vi "CG test stand DAQ main V2.vi"() -> ()   [LabVIEW 2020]
doc: "This example demonstrates how to read N channels of analog input from a LINX device."
uses:
  <vilib>/MakerHub/LINX/LMH-LINX.lvlib
  <vilib>/MakerHub/LINX/Public/Peripherals/Analog/Analog Read N Chans.vi
  <vilib>/MakerHub/LINX/Public/Utilities/Open Serial.vi
  <vilib>/Analysis/Matrix/NI_Matrix.lvlib
  <vilib>/Utility/file.llb/Write Delimited Spreadsheet (DBL).vi
  <vilib>/Analysis/Matrix/Numeric/Conversions/Array To Matrix - RA.vi
panel:
  in  "?":T1(tab)
  out "?":string
  out "?":string
  out "?":string
  out "?":string
  out "?":string
  out "?":string
  out "?":string
  out "?":dbl
  out "?":dbl
  out "?":dbl
  out "?":dbl
  out "?":dbl
  out "?":dbl
  out "?":dbl
  in  "Serial Port":refnum<visa-resource-name>
  in  "Filename":string
  in  "File extension":string
  in  "Path":path
  out "Full filepath":string
  out "error out":errorcluster
  out "?":dbl
  out "?":dbl
  out "?":dbl
  out "?":dbl
  out "?":dbl
  out "?":dbl
  out "?":dbl
  out "?":dbl
  out "?":dbl
  out "?":dbl
  out "?":dbl
  out "?":dbl
  out "?":dbl
  out "?":dbl
  out "?":dbl
  out "?":dbl
  out "?":dbl
  out "?":dbl
  out "?":dbl
  out "?":dbl
  out "?":dbl
  out "?":dbl
  out "?":dbl
  out "?":dbl
  out "?":dbl
  out "?":dbl
  out "?":dbl
  out "?":dbl
  out "?":dbl
  out "?":dbl
  out "?":dbl
  out "?":dbl
  out "?":dbl
  out "?":dbl
  out "?":dbl
  out "?":dbl
  out "?":dbl
  out "?":dbl
  out "?":dbl
  out "?":dbl
  out "?":dbl
  out "?":dbl
  out "?":dbl
  out "?":dbl
  out "?":dbl
  out "?":dbl
  out "?":dbl
  out "?":dbl
  out "?":dbl
  out "?":string
  out "?":dbl
  out "?":dbl
  out "?":dbl
  out "?":dbl
  out "?":dbl
  out "?":dbl
  out "?":dbl
  out "?":dbl
  out "?":dbl
  out "?":dbl
  out "?":dbl
  out "?":dbl
  out "?":dbl
  out "?":dbl
  out "?":string
  out "?":string
  out "?":dbl
  out "?":dbl
  out "?":dbl
  out "?":dbl
  out "?":dbl
  out "?":dbl
  out "?":dbl
  out "?":string
  out "?":dbl
  out "?":dbl
  out "?":dbl
  out "?":dbl
  out "?":dbl
  out "?":dbl
  out "?":dbl
  out "?":string
  in  "+      B":dbl
  in  "AX":dbl
  in  "Analog Port":dbl
  out "Time Stamp":timestamp
  out "Voltage":dbl
  out "Voltage":dbl(graph)
  out "Filtered Voltage":dbl(graph)
  out "Unfiltered Voltage":dbl
  out "Filtered Voltage":dbl
  out "Loop Rate (Hz)":u32
  in  "Stop Button":bool
  out "Pressure":dbl(graph)
  out "Pressure (PSI)":dbl
  out "WRITING TO FILE":bool
  in  "?":bool
  # "File Writing"
  # "Analog Inputs"
  # "Analog Port"
  # "Voltage In"
  # "X3"
  # "X2"
  # "X1"
  # "B"
  # "Instrument name"
  # "Scaled Value"
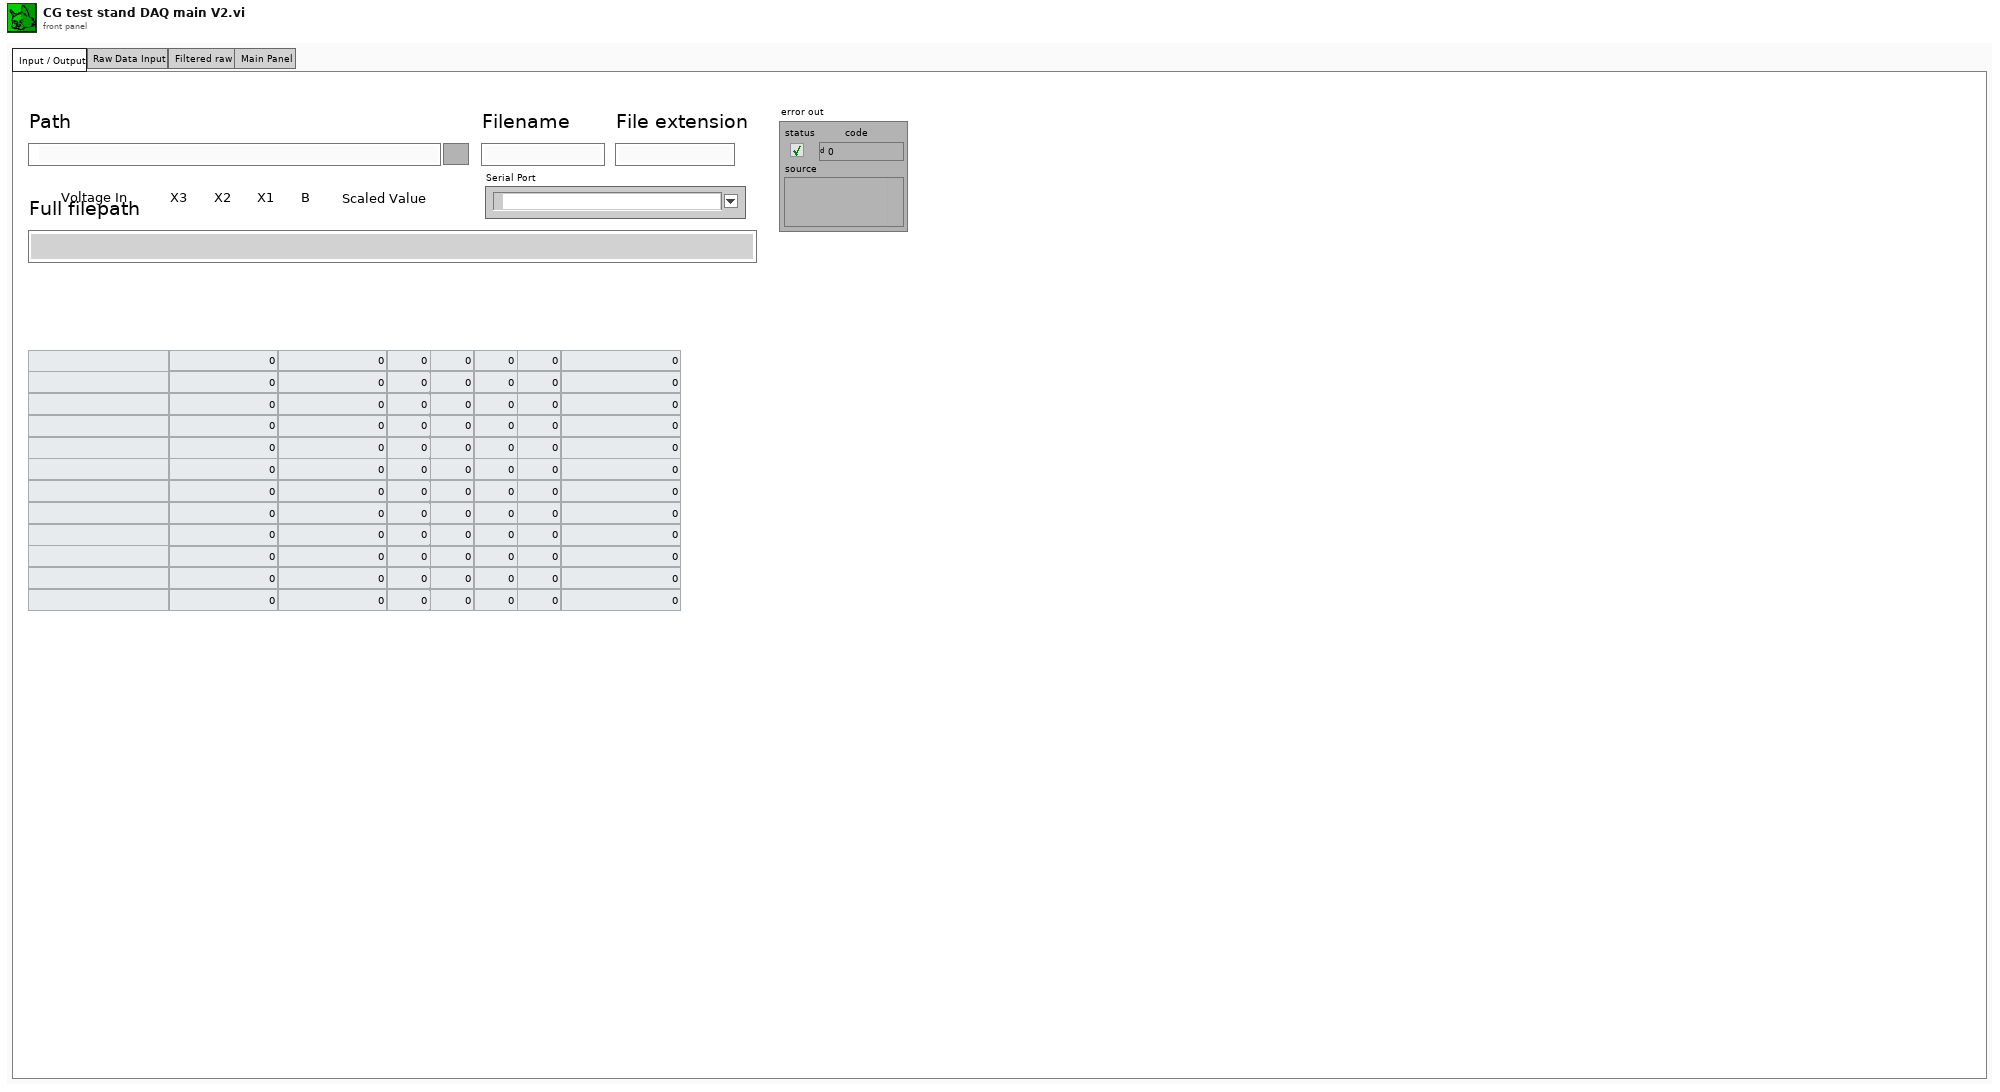
[diagram p1: front panel]
types:
  T1 = enum32{"Input / Output", "Raw Data Input", "Filtered raw", "Main Panel"}
  T2 = typedef "LMH-LINX.lvlib/LINX Ref.ctl" = cluster{"IO":T3, "Interface":T4, "LINX Device Config":T5}
  T3 = typedef "LMH-LINX.lvlib/Platform.ctl" = enum16{"Remote", "Local"}
  T4 = typedef "LMH-LINX.lvlib/Interface.ctl" = enum16{"Serial", "TCP"}
  T5 = typedef "LMH-LINX.lvlib/Device.lvlib/LINX Device Config.ctl" = cluster{"Interface":T4, "COM Port":refnum<visa-resource-name>, "TCP Configuration":T6, "Device Family":u8, "Device ID":u8, "Device Name":string, "TCP Ref":refnum<k5>, "Channels":T7}
  T6 = typedef "LMH-LINX.lvlib/Device.lvlib/TCP Config.ctl" = cluster{"IP Address":string, "Port":u16}
  T7 = typedef "LMH-LINX.lvlib/Channels.ctl" = cluster{"DI":u8[], "DO":u8[], "AI":u8[], "AO":u8[], "PWM":u8[], "QE":u8[], "UART":u8[], "I2C 2":u8[], "SPI":u8[], "CAN":u8[], "Servo":u8[], "AI Ref (V)":dbl, "AI Resolution (Bits)":u8, "AO Ref (V)":dbl, "AO Resolution (Bits)":u8}
  T8 = typedef "NI_Matrix.lvlib/RealMatrix.ctl" = dbl[][]
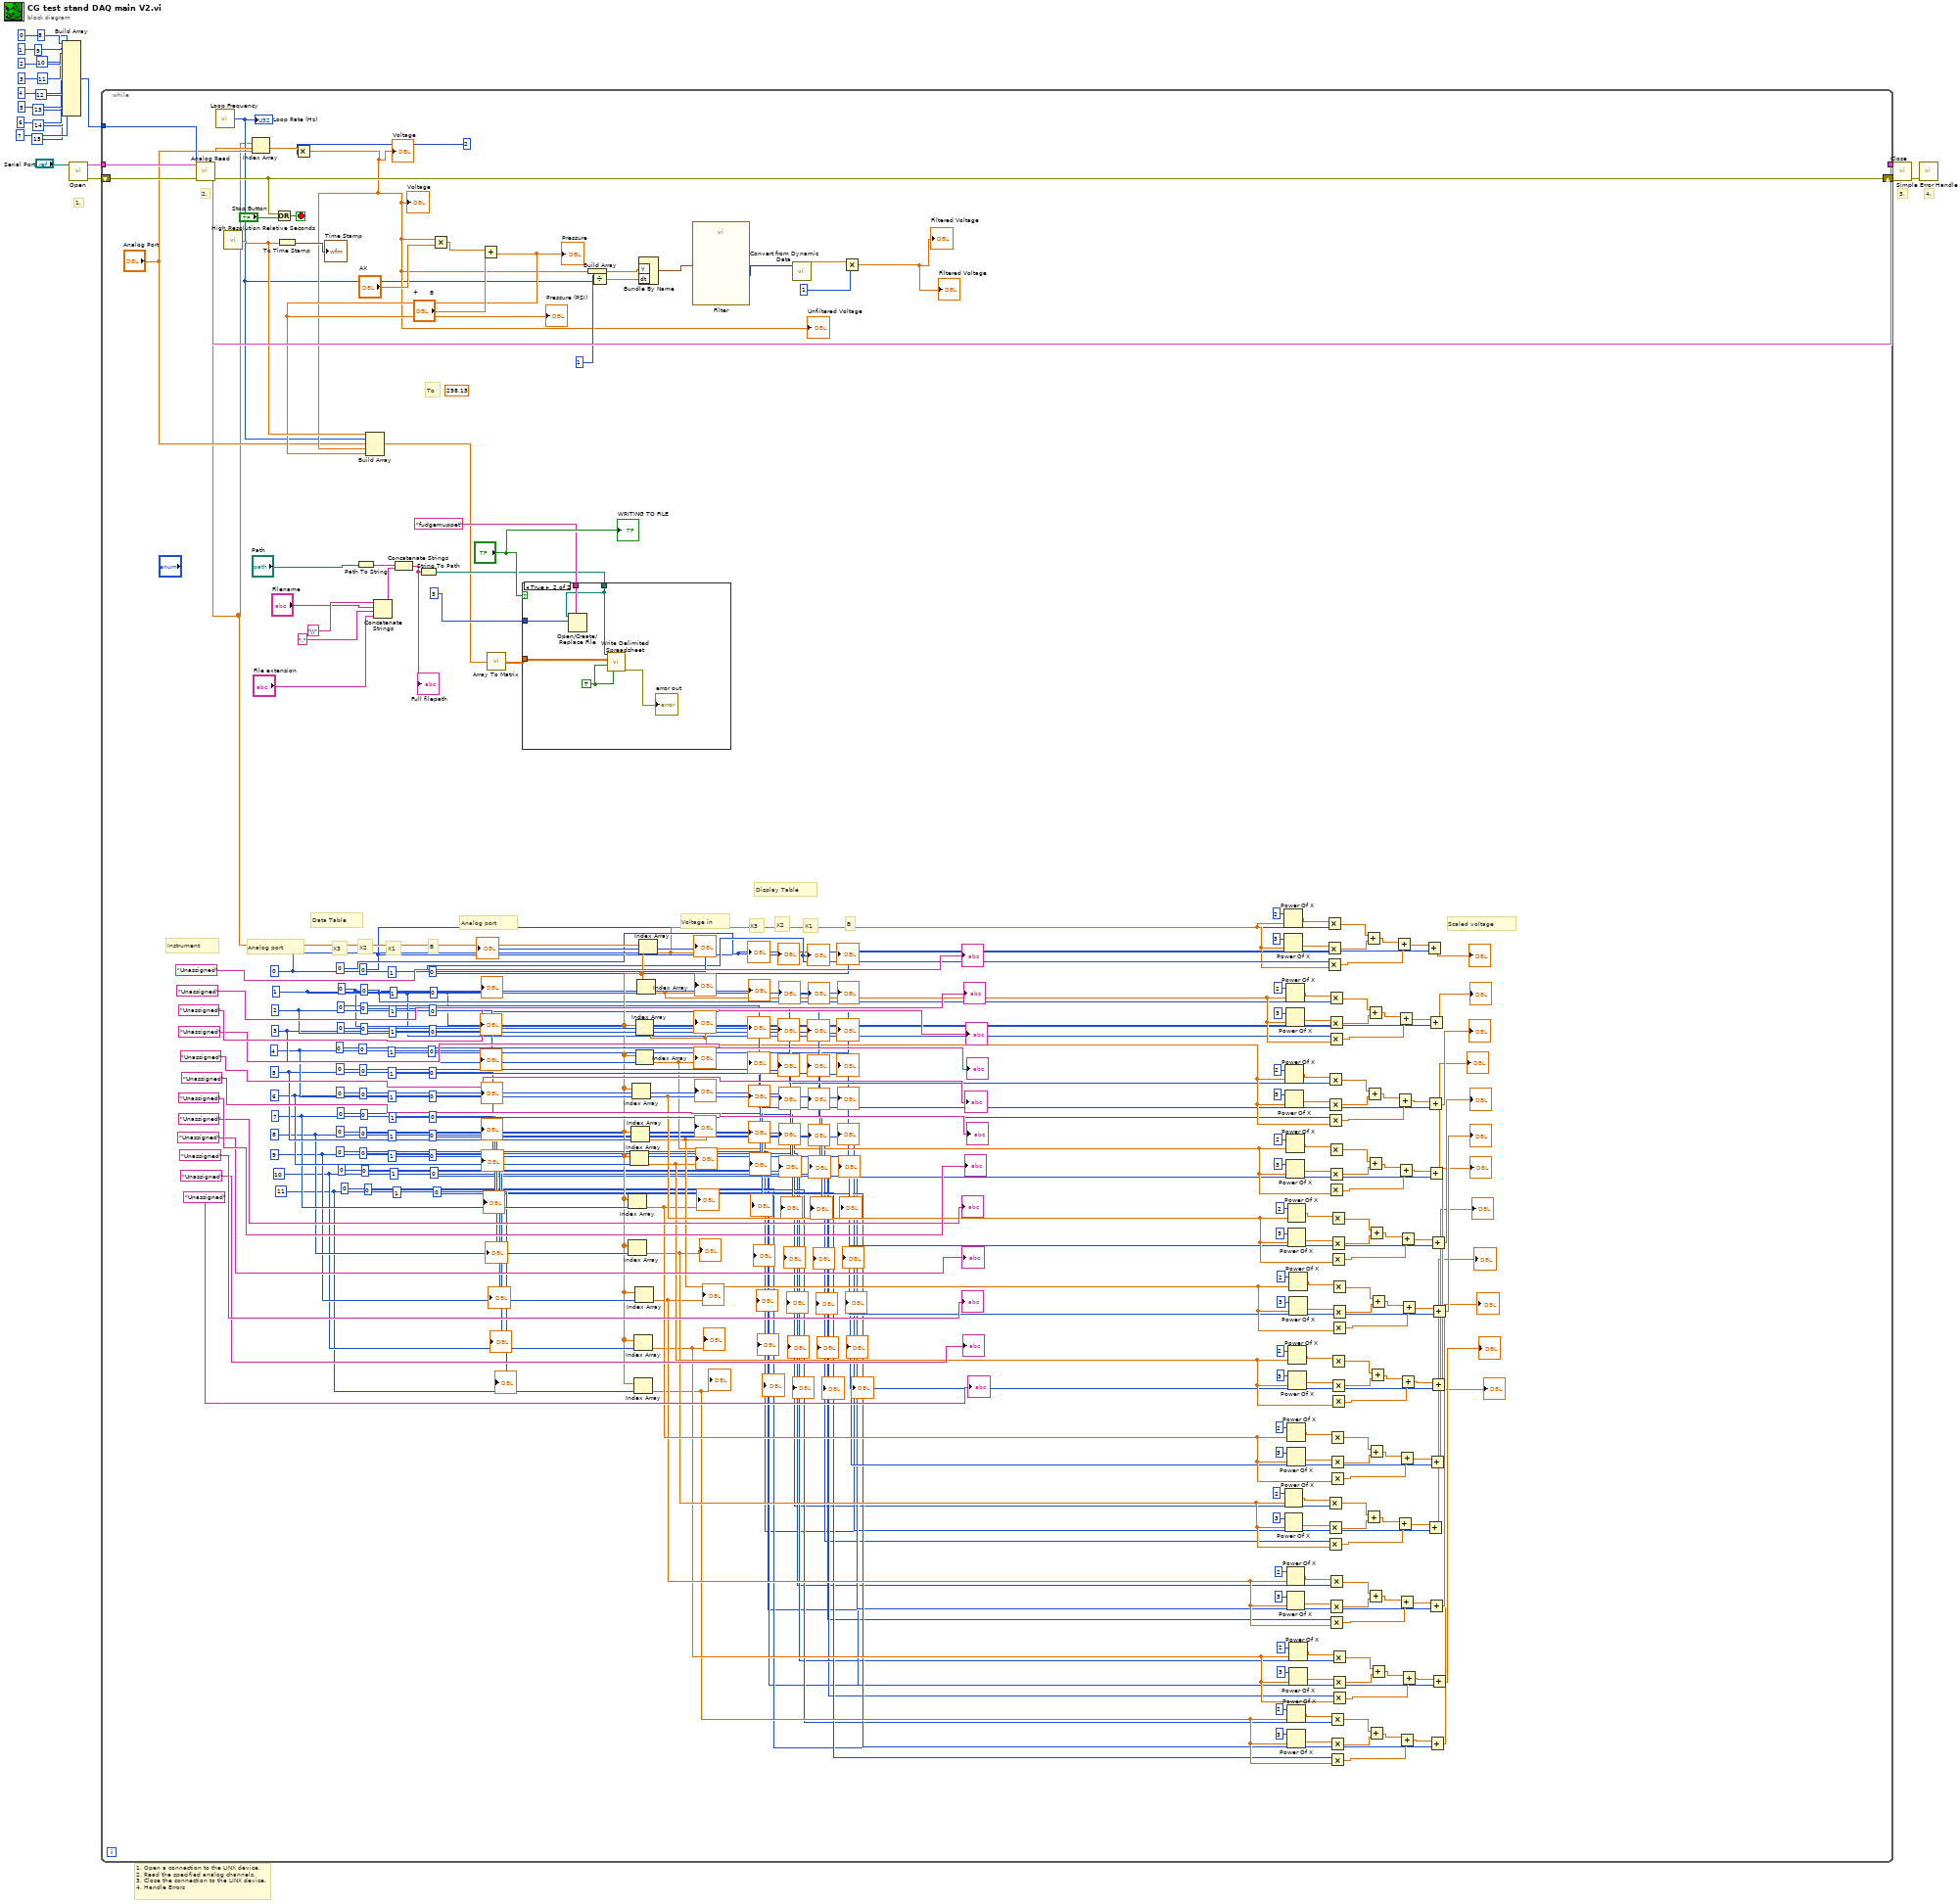
[diagram p0: block diagram]
diagram:
  # "1. Open a connection to the LINX device.\n2. Read the specified analog channels.\n3. Close the connection to the LINX device.\n4. Handle Errors"
  # "4."
  # "3."
  # "1."
  n1 = Build Array(0, 1, 2, 3, 4, 5, 6, 7, 8, 9, 10, 11, 12, 13, 14, 15) -> (w17:i32[])
  n2 = call-poly <vilib>:"Open.vi"("Serial Port"="Serial Port") -> ("Error Out"=w22:errorcluster, "LINX Resource"=w23:T2)  [unwired: 8 in, 1 out]
  n3 = while {
    tunnel: w23 -> [w268]
    tunnel: [w266] -> w21
    shift-right: [w263] -> w20
    shift-left: w22 -> [w267]
    tunnel: w17 -> [w262]
    stop <- w265 stop-if-true
    w39 = 0
    w36 = 1
    w35 = 0
    w34 = 0
    w70 = 11
    w33 = 0
    w31 = 1
    w32 = 0
    w30 = 0
    w71 = 10
    w38 = 0
    w29 = 1
    w28 = 0
    w27 = 0
    w72 = 9
    w37 = 0
    w26 = 1
    w25 = 0
    w24 = 0
    w73 = 8
    w40 = 0
    w74 = 7
    w41 = 0
    w75 = 6
    w42 = 0
    w76 = 5
    w43 = 0
    w77 = 4
    w44 = 0
    w78 = 3
    w45 = 0
    w48 = 1
    w50 = 0
    w49 = 0
    w79 = 2
    w46 = 0
    w51 = 1
    w53 = 0
    w52 = 0
    w80 = 1
    w47 = 0
    w57 = 1
    w54 = 0
    w56 = 0
    w81 = 0
    (unwired) 298.15
    # "Instrument"
    # "B"
    # "X3"
    # "X2"
    # "X1"
    # "Analog port"
    # "Data Table"
    # "Display Table"
    # "Voltage in"
    # "Scaled voltage"
    # "B"
    # "X3"
    # "X2"
    # "X1"
    # "Analog port"
    # "To"
    # "2."
    n4 = call-poly <vilib>:"Analog Read.vi"("Error In"=w267, "AI Channel(s)"=w262, "LINX Resource"=w268) -> ("Error Out"=w263:errorcluster, "Voltages"=w69:dbl[], "LINX Resource"=w266:T2)  [unwired: 5 in, 1 out]
    n5 = call <vilib>:"Loop Frequency.vi"() -> ("Loop Rate (Hz)"=w243:u32)
    "Loop Rate (Hz)" <- w243
    n6 = call <vilib>:"High Resolution Relative Seconds.vi"() -> ("relative seconds"=w257:dbl)
    n7 = Index Array(array=w69, index="Analog Port") -> (element=w252:dbl)
    n8 = Or(x=w263, y="Stop Button") -> (x .or. y?=w265:bool)
    n9 = To Time Stamp(1:w257) -> (0:→"Time Stamp":timestamp)
    n10 = Multiply(x=w252, y=2) -> (x*y=w245:dbl)
    "Voltage" <- w245
    "Voltage" <- w245
    "Unfiltered Voltage" <- w245
    n11 = Path To String(path="Path") -> (string=w236:string)
    n12 = Concatenate Strings("\\", "Filename", ".", "File extension") -> (w229:string)
    n13 = Concatenate Strings(w236, w229) -> (w237:string)
    "Full filepath" <- w237
    n14 = String To Path(string=w237) -> (path=w238:path)
    n15 = Multiply(x=w245, y="AX") -> (x*y=w259:dbl)
    n16 = Add(x=w259, y="+      B") -> (x+y=w246:dbl)
    "Pressure" <- w246
    "Pressure (PSI)" <- w246
    n17 = Build Array(w257, w243, "Analog Port", w245, w246) -> (w234:dbl[])
    n18 = call-poly <vilib>:"Array To Matrix.vi"("Real 1D Array"=w234) -> ("Real Matrix (Column Vector)"=w242:T8)
    n19 = case shown="True" "?" {
      tunnel: w238 -> [_ w272]
      tunnel: w242 -> [_ w269]
      tunnel: "fudgemuppet" -> [_ w274]
      tunnel: 3 -> [_ w273]
      frame False {
      }
      frame True {
        w270 = TRUE
        n20 = Open/Create/Replace File(file path (use dialog)=w272, prompt=w274, operation (0:open)=w273) -> ()  [unwired: 3 in, 3 out]
        n21 = call-poly <vilib>:"Write Delimited Spreadsheet.vi"("file path (dialog if empty)"=w272, "2D data"=w269, "append to file? (new file:F)"=w270, "transpose? (no:F)"=w270) -> ("error out"=→"error out":errorcluster)  [unwired: 10 in, 1 out]
      }
    }
    n22 = Build Array(w245) -> (w254:dbl[])
    n23 = Divide(x=1, y=w243) -> (x/y=w256:dbl)
    n24 = Index Array(array=w69, index=w73) -> (element=w61:dbl)
    "?" <- w61
    n25 = Index Array(array=w69, index=w74) -> (element=w62:dbl)
    "?" <- w62
    n26 = Index Array(array=w69, index=w75) -> (element=w63:dbl)
    "?" <- w63
    n27 = Index Array(array=w69, index=w76) -> (element=w64:dbl)
    "?" <- w64
    n28 = Index Array(array=w69, index=w77) -> (element=w65:dbl)
    "?" <- w65
    n29 = Index Array(array=w69, index=w71) -> (element=w59:dbl)
    "?" <- w59
    n30 = Index Array(array=w69, index=w70) -> (element=w58:dbl)
    "?" <- w58
    n31 = Index Array(array=w69, index=w72) -> (element=w60:dbl)
    "?" <- w60
    n32 = Index Array(array=w69, index=w79) -> (element=w67:dbl)
    "?" <- w67
    n33 = Index Array(array=w69, index=w78) -> (element=w66:dbl)
    "?" <- w66
    n34 = Index Array(array=w69, index=w80) -> (element=w68:dbl)
    "?" <- w68
    n35 = Bundle By Name("Y"=w254, "dt"=w256) -> (w253:waveform(dbl))  [unwired: 1 in]
    n36 = Index Array(array=w69, index=w81) -> (element=w55:dbl)
    "?" <- w55
    n37 = call "Filter"("Signal"=w253) -> ("Filtered Signal"=w250:dynamicdata)  [unwired: 9 in, 1 out]
    n38 = call "Convert from Dynamic Data"("Dynamic Data Type"=w250) -> ("Scalar"=w249:dbl)  [unwired: 3 in]
    n39 = Multiply(x=w249, y=1) -> (x*y=→"Filtered Voltage" →"Filtered Voltage":dbl)
    n40 = Power Of X(1:w55, 2:2) -> (0:w201:dbl)
    n41 = Power Of X(1:w55, 2:3) -> (0:w198:dbl)
    n42 = Power Of X(1:w61, 2:2) -> (0:w129:dbl)
    n43 = Power Of X(1:w61, 2:3) -> (0:w126:dbl)
    n44 = Power Of X(1:w67, 2:2) -> (0:w183:dbl)
    n45 = Power Of X(1:w67, 2:3) -> (0:w180:dbl)
    n46 = Power Of X(1:w68, 2:2) -> (0:w192:dbl)
    n47 = Power Of X(1:w68, 2:3) -> (0:w189:dbl)
    n48 = Power Of X(1:w66, 2:2) -> (0:w174:dbl)
    n49 = Power Of X(1:w66, 2:3) -> (0:w171:dbl)
    n50 = Power Of X(1:w60, 2:2) -> (0:w120:dbl)
    n51 = Power Of X(1:w60, 2:3) -> (0:w117:dbl)
    n52 = Power Of X(1:w62, 2:2) -> (0:w138:dbl)
    n53 = Power Of X(1:w62, 2:3) -> (0:w135:dbl)
    n54 = Power Of X(1:w58, 2:2) -> (0:w102:dbl)
    n55 = Power Of X(1:w58, 2:3) -> (0:w99:dbl)
    n56 = Power Of X(1:w65, 2:2) -> (0:w165:dbl)
    n57 = Power Of X(1:w65, 2:3) -> (0:w162:dbl)
    n58 = Power Of X(1:w63, 2:2) -> (0:w147:dbl)
    n59 = Power Of X(1:w63, 2:3) -> (0:w144:dbl)
    n60 = Power Of X(1:w64, 2:2) -> (0:w156:dbl)
    n61 = Power Of X(1:w64, 2:3) -> (0:w153:dbl)
    n62 = Power Of X(1:w59, 2:2) -> (0:w111:dbl)
    n63 = Power Of X(1:w59, 2:3) -> (0:w108:dbl)
    n64 = Multiply(x=w201, y=w54) -> (x*y=w196:dbl)
    n65 = Multiply(x=w198, y=w56) -> (x*y=w197:dbl)
    n66 = Multiply(x=w57, y=w55) -> (x*y=w194:dbl)
    n67 = Multiply(x=w129, y=w25) -> (x*y=w124:dbl)
    n68 = Multiply(x=w126, y=w24) -> (x*y=w125:dbl)
    n69 = Multiply(x=w26, y=w61) -> (x*y=w122:dbl)
    n70 = Multiply(x=w183, y=w50) -> (x*y=w178:dbl)
    n71 = Multiply(x=w180, y=w49) -> (x*y=w179:dbl)
    n72 = Multiply(x=w48, y=w67) -> (x*y=w176:dbl)
    n73 = Multiply(x=w192, y=w53) -> (x*y=w187:dbl)
    n74 = Multiply(x=w189, y=w52) -> (x*y=w188:dbl)
    n75 = Multiply(x=w51, y=w68) -> (x*y=w185:dbl)
    n76 = Multiply(x=w174) -> (x*y=w169:dbl)  [unwired: 1 in]
    n77 = Multiply(x=w171) -> (x*y=w170:dbl)  [unwired: 1 in]
    n78 = Multiply(y=w66) -> (x*y=w167:dbl)  [unwired: 1 in]
    n79 = Multiply(x=w120, y=w28) -> (x*y=w115:dbl)
    n80 = Multiply(x=w117, y=w27) -> (x*y=w116:dbl)
    n81 = Multiply(x=w29, y=w60) -> (x*y=w113:dbl)
    n82 = Multiply(x=w138) -> (x*y=w133:dbl)  [unwired: 1 in]
    n83 = Multiply(x=w135) -> (x*y=w134:dbl)  [unwired: 1 in]
    n84 = Multiply(y=w62) -> (x*y=w131:dbl)  [unwired: 1 in]
    n85 = Multiply(x=w102, y=w35) -> (x*y=w97:dbl)
    n86 = Multiply(x=w99, y=w34) -> (x*y=w98:dbl)
    n87 = Multiply(x=w36, y=w58) -> (x*y=w95:dbl)
    n88 = Multiply(x=w165) -> (x*y=w160:dbl)  [unwired: 1 in]
    n89 = Multiply(x=w162) -> (x*y=w161:dbl)  [unwired: 1 in]
    n90 = Multiply(y=w65) -> (x*y=w158:dbl)  [unwired: 1 in]
    n91 = Multiply(x=w147) -> (x*y=w142:dbl)  [unwired: 1 in]
    n92 = Multiply(x=w144) -> (x*y=w143:dbl)  [unwired: 1 in]
    n93 = Multiply(y=w63) -> (x*y=w140:dbl)  [unwired: 1 in]
    n94 = Multiply(x=w156) -> (x*y=w151:dbl)  [unwired: 1 in]
    n95 = Multiply(x=w153) -> (x*y=w152:dbl)  [unwired: 1 in]
    n96 = Multiply(y=w64) -> (x*y=w149:dbl)  [unwired: 1 in]
    n97 = Multiply(x=w111, y=w32) -> (x*y=w106:dbl)
    n98 = Multiply(x=w108, y=w30) -> (x*y=w107:dbl)
    n99 = Multiply(x=w31, y=w59) -> (x*y=w104:dbl)
    n100 = Add(x=w196, y=w197) -> (x+y=w195:dbl)
    n101 = Add(x=w124, y=w125) -> (x+y=w123:dbl)
    n102 = Add(x=w178, y=w179) -> (x+y=w177:dbl)
    n103 = Add(x=w187, y=w188) -> (x+y=w186:dbl)
    n104 = Add(x=w169, y=w170) -> (x+y=w168:dbl)
    n105 = Add(x=w115, y=w116) -> (x+y=w114:dbl)
    n106 = Add(x=w133, y=w134) -> (x+y=w132:dbl)
    n107 = Add(x=w97, y=w98) -> (x+y=w96:dbl)
    n108 = Add(x=w160, y=w161) -> (x+y=w159:dbl)
    n109 = Add(x=w142, y=w143) -> (x+y=w141:dbl)
    n110 = Add(x=w151, y=w152) -> (x+y=w150:dbl)
    n111 = Add(x=w106, y=w107) -> (x+y=w105:dbl)
    n112 = Add(x=w195, y=w194) -> (x+y=w193:dbl)
    n113 = Add(x=w123, y=w122) -> (x+y=w121:dbl)
    n114 = Add(x=w177, y=w176) -> (x+y=w175:dbl)
    n115 = Add(x=w186, y=w185) -> (x+y=w184:dbl)
    n116 = Add(x=w168, y=w167) -> (x+y=w166:dbl)
    n117 = Add(x=w114, y=w113) -> (x+y=w112:dbl)
    n118 = Add(x=w132, y=w131) -> (x+y=w130:dbl)
    n119 = Add(x=w96, y=w95) -> (x+y=w94:dbl)
    n120 = Add(x=w159, y=w158) -> (x+y=w157:dbl)
    n121 = Add(x=w141, y=w140) -> (x+y=w139:dbl)
    n122 = Add(x=w150, y=w149) -> (x+y=w148:dbl)
    n123 = Add(x=w105, y=w104) -> (x+y=w103:dbl)
    n124 = Add(x=w193, y=w47) -> (x+y=→"?":dbl)
    n125 = Add(x=w121, y=w37) -> (x+y=→"?":dbl)
    n126 = Add(x=w175, y=w45) -> (x+y=→"?":dbl)
    n127 = Add(x=w184, y=w46) -> (x+y=→"?":dbl)
    n128 = Add(x=w166, y=w44) -> (x+y=→"?":dbl)
    n129 = Add(x=w112, y=w38) -> (x+y=→"?":dbl)
    n130 = Add(x=w130, y=w40) -> (x+y=→"?":dbl)
    n131 = Add(x=w94, y=w39) -> (x+y=→"?":dbl)
    n132 = Add(x=w157, y=w43) -> (x+y=→"?":dbl)
    n133 = Add(x=w139, y=w41) -> (x+y=→"?":dbl)
    n134 = Add(x=w148, y=w42) -> (x+y=→"?":dbl)
    n135 = Add(x=w103, y=w33) -> (x+y=→"?":dbl)
    "WRITING TO FILE" <- "?"
    "?" <- w81
    "?" <- w56
    "?" <- w54
    "?" <- w57
    "?" <- w47
    "?" <- w80
    "?" <- w52
    "?" <- w53
    "?" <- w51
    "?" <- w46
    "?" <- w79
    "?" <- w49
    "?" <- w50
    "?" <- w48
    "?" <- w45
    "?" <- w78
    "?" <- 0
    "?" <- 0
    "?" <- 1
    "?" <- w44
    "?" <- w77
    "?" <- 0
    "?" <- 0
    "?" <- 1
    "?" <- w43
    "?" <- w76
    "?" <- 0
    "?" <- 0
    "?" <- 1
    "?" <- w42
    "?" <- w75
    "?" <- 0
    "?" <- 0
    "?" <- 1
    "?" <- w41
    "?" <- w74
    "?" <- 0
    "?" <- 0
    "?" <- 1
    "?" <- w40
    "?" <- "Unassigned"
    "?" <- "Unassigned"
    "?" <- "Unassigned"
    "?" <- "Unassigned"
    "?" <- "Unassigned"
    "?" <- w73
    "?" <- w24
    "?" <- w25
    "?" <- w26
    "?" <- w37
    "?" <- w72
    "?" <- w27
    "?" <- w28
    "?" <- w29
    "?" <- w38
    "?" <- "Unassigned"
    "?" <- "Unassigned"
    "?" <- "Unassigned"
    "?" <- "Unassigned"
    "?" <- "Unassigned"
    "?" <- w71
    "?" <- w30
    "?" <- w32
    "?" <- w31
    "?" <- w33
    "?" <- "Unassigned"
    "?" <- w70
    "?" <- w34
    "?" <- w35
    "?" <- w36
    "?" <- w39
    "?" <- "Unassigned"
  }
  n136 = call <vilib>:"Close.vi"("Error In"=w20, "LINX Resource"=w21) -> ("Error Out"=w18:errorcluster)  [unwired: 9 in]
  n137 = call <vilib>:"Simple Error Handler.vi"("error in (no error)"=w18) -> ()  [unwired: 4 in, 5 out]
